vi "Generate Task ID_IO.vi"(8 "error in (no error)":errorcluster) -> (0 "error out":errorcluster, 3 "Task ID":string)   [LabVIEW 2022 SP3, in "IO.lvclass"]
uses:
  IO.lvclass
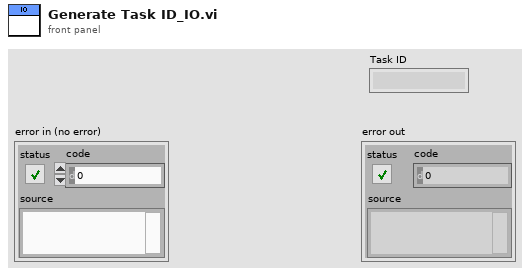
[diagram p1: front panel]
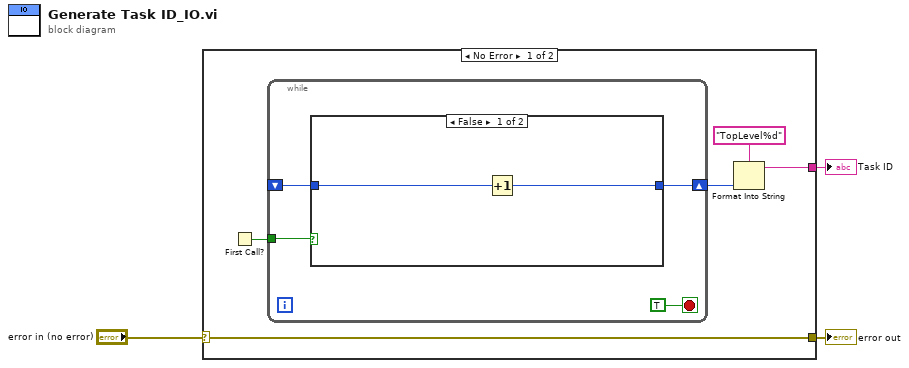
[diagram p0: block diagram]
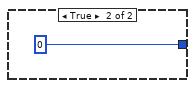
[diagram p2: hidden frame]
diagram:
  n1 = case shown="No Error" "error in (no error)" {
    selector: "error in (no error)" -> [w7 w16]
    tunnel: [w7 w16] -> w2
    tunnel: [w4 _] -> w1
    frame No Error {
      n2 = First Call?() -> (First Call?: T/F=w8:bool)
      n3 = while {
        tunnel: w8 -> [w11]
        shift-right: [w10] -> w6
        shift-left: _ -> [w9]
        stop <- TRUE stop-if-true
        n4 = case shown="False" w11 {
          tunnel: [w13 0] -> w10
          tunnel: w9 -> [w14 _]
          frame False {
            n5 = Increment(x=w14) -> (x+1=w13:i32)
          }
          frame True {
          }
        }
      }
      n6 = Format Into String(format string="TopLevel%d", w6) -> (resulting string=w4:string)  [unwired: 2 in, 1 out]
    }
    frame Error {
    }
  }
  "error out" <- w2
  "Task ID" <- w1
